vi "Write Read Multi Test.vi"(8 "error in (no error)":errorcluster, 10 "Test Value":dbl[](array[numeric]) format="%#_12g", 11 "Type":T1=enum."Double Float") -> (0 "error out":errorcluster)   [LabVIEW 2021]
uses:
  <vilib>/Utility/Data Type/Type Definitions/Data Type.ctl
  Source/Omni-Bus/Omni_Bus.lvclass
  Source/Local Bus/Local Bus.lvclass
  C:/TSA/Omni-Bus/Source/Omni-Bus/Bus Access/Bus_Access.lvclass
  <vilib>/TSA/Abstract Data Classes/Abs_Types/Type/Abs_Type.lvclass/Abs_Type.ctl
  Source/Omni-Bus/Omni_Bus.lvclass/Omni_Bus.ctl
  Source/Omni-Bus/Support/Get/Get Multi EXT.vi
  Source/Omni-Bus/Support/FindMultiVar.vi
  Source/Omni-Bus/Support/FindVar.vi
  <vilib>/Utility/error.llb/Clear Errors.vi
  <vilib>/TSA/Abstract Data Classes/Abs_Types/Type/Properties/Write Tag.vi
  Source/Omni-Bus/Properties/Read Var Map.vi
  <vilib>/TSA/Abstract Data Classes/Abs_Types/Type/Properties/Read Tag.vi
  <vilib>/TSA/Abstract Data Classes/Abs_Types/Extended Float/Abs_Extended Float.lvclass
  C:/Program Files (x86)/National Instruments/LabVIEW 2021/vi.lib/TSA/Abstract Data Classes/Abs_Types/Type/Abs_Type.lvclass
  <vilib>/TSA/Abstract Data Classes/Abs_Types/Value/Abs_Value.lvclass
  Source/Omni-Bus/Support/Check For Read Only Error.vi
  Source/Omni-Bus/Support/Incorrect Tag String Error.vi
  <vilib>/TSA/Abstract Data Classes/Abs_Types/Type/Abs_Type.lvclass
  <vilib>/Utility/Data Type/NI_Data Type.lvlib
  <vilib>/addons/_JKI Toolkits/Caraya/classes/Assert/Assert.lvclass
  <vilib>/addons/_JKI Toolkits/Caraya/classes/Test/Test.lvclass
  <vilib>/addons/_JKI Toolkits/Caraya/classes/Assert/Assert Equal Value_Variant.vi
  <vilib>/addons/_JKI Toolkits/Caraya/classes/Assert/Assert Not Error.vi
  Source/Omni-Bus/Support/Write/Write Multi DBL.vi
  Source/Omni-Bus/Support/Read/Read Multi DBL.vi
panel:
  out "Numeric":dbl[](array[numeric]) format="%#_15g"
  out "Test Value 2":dbl[](array[numeric]) format="%#_15g"
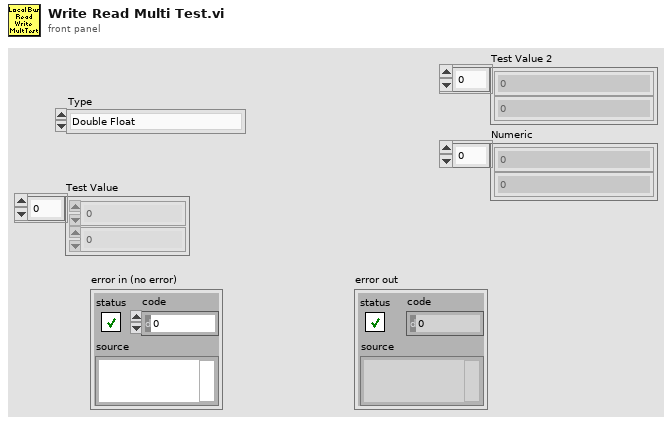
[diagram p1: front panel]
types:
  T1 = typedef "NI_Data Type.lvlib/Data Type.ctl" = enum8{"Invalid Type", "Void", "I8", "I16", "I32", "I64", "U8", "U16", "U32", "U64", "Single Float", "Double Float", "Extended Float", "Single Complex", "Double Complex", "Extended Complex", "Enum U8", "Enum U16", "Enum U32", "Enum U64", "Single Float With Unit", "Double Float With Unit", "Extended Float With Unit", "Single Complex with Unit", "Double Complex with Unit", "Extended Complex with Unit", "Boolean", "String", "Path", "Picture", "Tag", "Array", "Cluster", "Variant", "LV Variant", "Waveform", "Timestamp", "Digital Waveform", "Digital Data", "ExpressData", "Refnum", "External Data", "VI", "Poly VI", "LabVIEW Class Instance", "Fixed Point", "Set Collection", "Map Collection"}
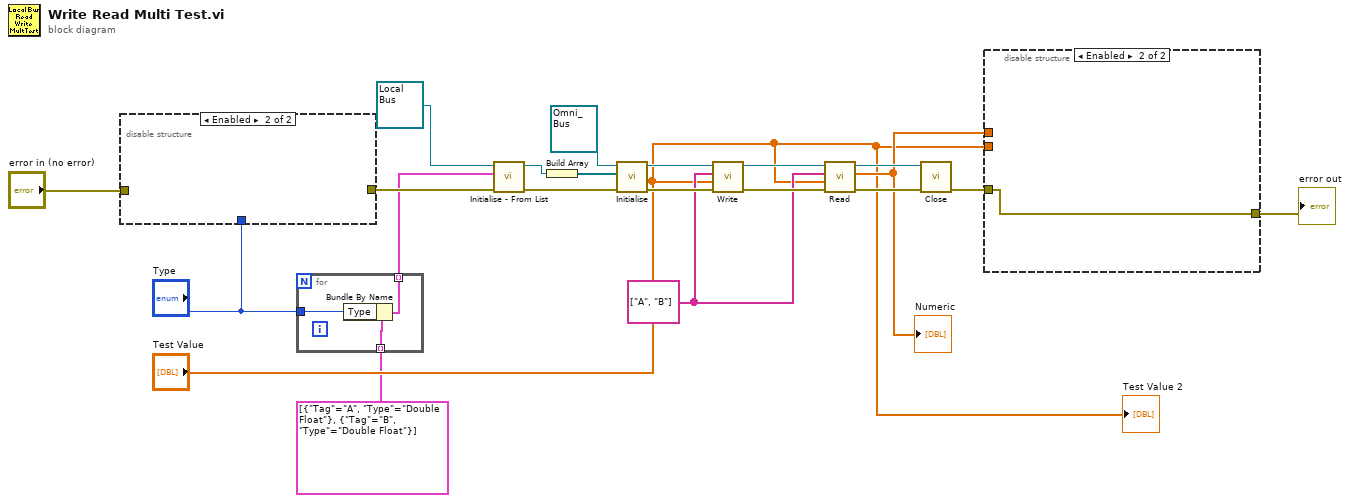
[diagram p0: block diagram]
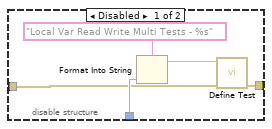
[diagram p2: hidden frame]
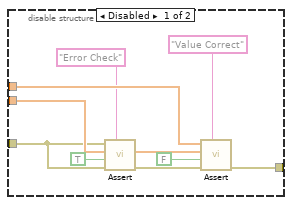
[diagram p3: hidden frame]
diagram:
  w12 = string[] ["A", "B"] ("Tag")
  n1 = disable-structure shown="Enabled" {
    disable-tunnel: "Type" -> [w26 _]
    disable-tunnel: [w24 _] -> w5
    disable-tunnel: "error in (no error)" -> [w23 _]
    frame Disabled {
      n2 = Format Into String(format string="Local Var Read Write Multi Tests - %s", w26) -> (resulting string=w22:string)  [unwired: 2 in, 1 out]
      n3 = call <vilib>:"Define Test.vi"("error in (no error)"=w23, "Label (VI Title)"=w22) -> ("error out"=w24:errorcluster)  [unwired: 8 in, 1 out]
    }
    frame Enabled {
    }
  }
  n4 = for {
    tunnel: "Type" -> [w29]
    tunnel: cluster{"Tag":string, "Type":T1}[] [{"Tag"="A", "Type"=enum."Double Float"}, {"Tag"="B", "Type"=enum."Double Float"}] ("Cluster") -> [w28] mode=indexing
    tunnel: [w27] -> w1 mode=indexing
    n5 = Bundle By Name(cluster=w28, "Type"=w29) -> (w27:cluster{"Tag":string, "Type":T1})
  }
  n6 = call "Initialise - From List.vi"("error in (no error)"=w5, "Tag List"=w1, "Local Bus in"=refnum<class "Local Bus.lvclass"> refnum ("Local Bus.lvclass")) -> ("error out"=w19:errorcluster, "Local Bus out"=w20:refnum<class "Local Bus.lvclass">)  [unwired: 7 in]
  n7 = Build Array(w20) -> (w18:refnum<class "Local Bus.lvclass">[])
  n8 = call-dynamic "Initialise.vi"("error in (no error)"=w19, "Bus Access"=w18, "Var Bus in"=refnum<class "Omni_Bus.lvclass"> refnum) -> ("error out"=w13:errorcluster, "Var Bus out"=w14:refnum<class "Omni_Bus.lvclass">)  [unwired: 7 in]
  n9 = call-poly "Write.vi"("error in (no error)"=w13, "Array"="Test Value", "Tag"=w12, "Omni_Bus in"=w14) -> ("error out"=w16:errorcluster, "Omni_Bus out"=w15:refnum<class "Omni_Bus.lvclass">)  [unwired: 6 in]
  n10 = call-poly "Read.vi"("error in (no error)"=w16, "Type"="Test Value", "Tag"=w12, "Var Bus in"=w15) -> ("error out"=w10:errorcluster, "DBL's"=w9:dbl[], "Var Bus out"=w11:refnum<class "Omni_Bus.lvclass">)  [unwired: 5 in]
  "Numeric" <- w9
  n11 = call-dynamic "Close.vi"("error in (no error)"=w10, "Data in"=w11) -> ("error out"=w3:errorcluster)  [unwired: 8 in, 1 out]
  n12 = disable-structure shown="Enabled" {
    disable-tunnel: w9 -> [w38 _]
    disable-tunnel: "Test Value" -> [w37 _]
    disable-tunnel: [w35 w39] -> w7
    disable-tunnel: w3 -> [w32 w39]
    frame Disabled {
      n13 = call-poly <vilib>:"Assert.vi"("Label"="Error Check", "error in (no error)"=w32, "Register with caller test (F)"=TRUE, "Not Error?"=w32) -> ("error out"=w36:errorcluster)  [unwired: 6 in, 1 out]
      n14 = call-poly <vilib>:"Assert.vi"("Label"="Value Correct", "error in (no error)"=w36, "Register with caller test (F)"=FALSE, "Actual"=w37, "Expected"=w38) -> ("error out"=w35:errorcluster)  [unwired: 5 in, 1 out]
    }
    frame Enabled {
    }
  }
  "error out" <- w7
  "Test Value 2" <- "Test Value"
